vi "Script_Extract_Waveforms.vi"(8 "error in (no error)":errorcluster, 9 "Script File":string="Adiabatic.txt", 10 "Script Path":path=path "D:/PIRENEA/SEQUENCE_SCRIPTS") -> (0 "error out":errorcluster, 3 "Table of Waveforms":string[](array[string]))   [LabVIEW 2015]
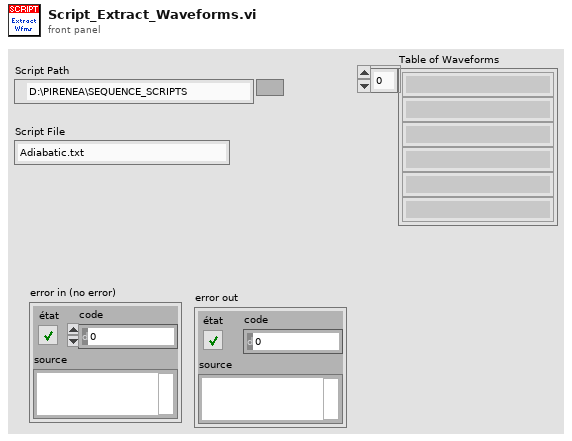
[diagram p1: front panel]
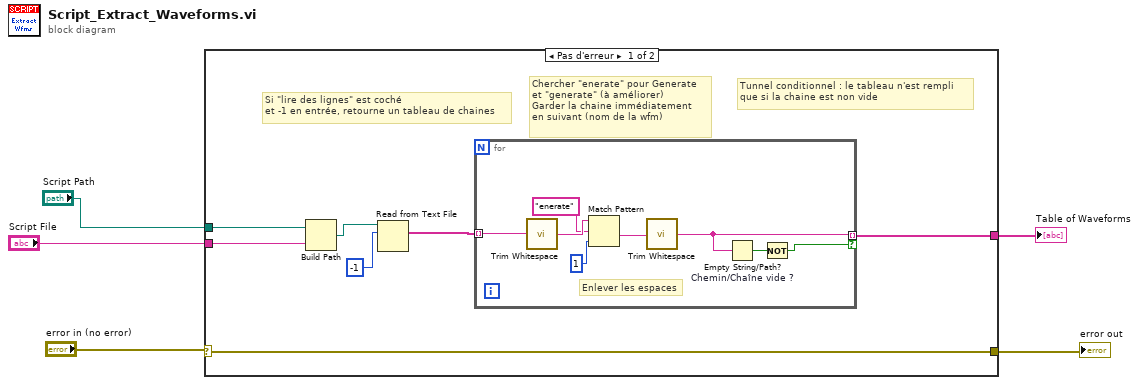
[diagram p0: block diagram]
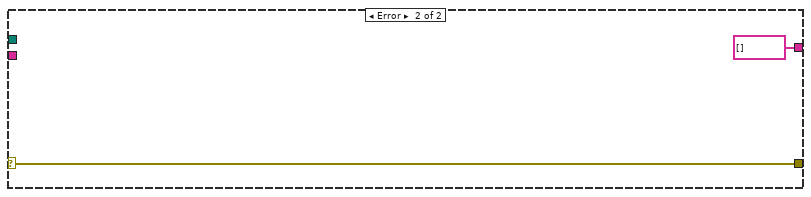
[diagram p2: hidden frame]
diagram:
  n1 = case shown="Pas d'erreur" "error in (no error)" {
    selector: "error in (no error)" -> [w9 w22]
    tunnel: "Script File" -> [w12 _]
    tunnel: [w9 w22] -> w3
    tunnel: "Script Path" -> [w11 _]
    tunnel: [w6 string[] []] -> w1
    frame No Error {
      # "Tunnel conditionnel : le tableau n'est rempli\nque si la chaine est non vide"
      # "Chercher \"enerate\" pour Generate\net \"generate\" (à améliorer)\nGarder la chaine immédiatement\nen suivant (nom de la wfm)"
      # "Si \"lire des lignes\" est coché\net -1 en entrée, retourne un tableau de chaines"
      n2 = Build Path(base path=w11, name or relative path=w12) -> (appended path=w10:path)
      n3 = Read from Text File(file (use dialog)=w10, count=-1 ("nombre")) -> (text=w7:string[])  [unwired: 2 in, 3 out]
      n4 = for {
        tunnel: w7 -> [w20] mode=indexing
        tunnel: [w13] -> w6 mode=indexing if=w14
        # "Enlever les espaces"
        n5 = call <vilib>:"Trim Whitespace.vi"("string"=w20) -> ("trimmed string"=w19:string)  [unwired: 1 in]
        n6 = Match Pattern(string=w19, regular expression="enerate" ("expression régulière"), offset (0)=1) -> (after substring=w16:string)  [unwired: 3 out]
        n7 = call <vilib>:"Trim Whitespace.vi"("string"=w16) -> ("trimmed string"=w13:string)  [unwired: 1 in]
        n8 = Empty String/Path? "Chemin/Chaîne vide ?"(string/path=w13) -> (empty?=w15:bool)
        n9 = Not(x=w15) -> (.not. x?=w14:bool)
      }
    }
    frame Error {
    }
  }
  "error out" <- w3
  "Table of Waveforms" <- w1
